vi "Set temperature.vi"(8 "error in (no error)":errorcluster, 9 "Heater":T1, 10 "Temperature":i32, 11 "VISA resource name":refnum<visa-resource-name>) -> (0 "error out":errorcluster, 3 "VISA resource name out":refnum<visa-resource-name>)   [LabVIEW 2020, in "Marlin Instrument Driver.lvlib"]
doc: "Returns the current state of the configured X, Y, Z endstops. Takes into account any 'inverted endstop' settings, so one can confirm that the machine is interpreting the endstops correctly."
uses:
  <instrlib>/Marlin Instrument Driver/Marlin Instrument Driver.lvlib
  <instrlib>/Marlin Instrument Driver/Public/controls/heater.ctl
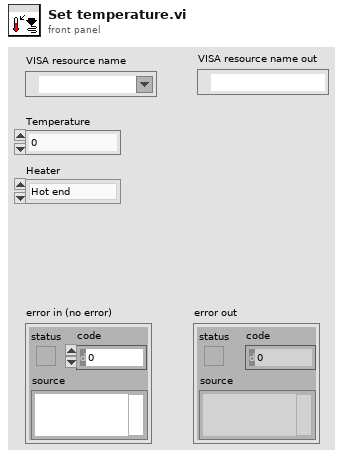
[diagram p1: front panel]
types:
  T1 = typedef "Marlin Instrument Driver.lvlib/heater.ctl" = enum16{"Hot end", "Bed", "Chamber"}
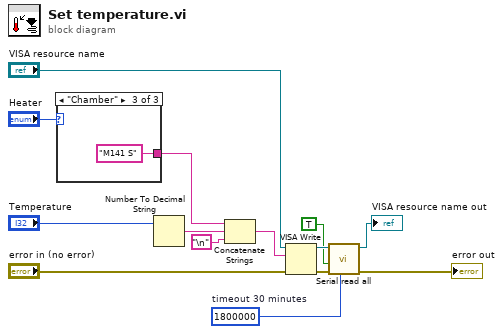
[diagram p0: block diagram]
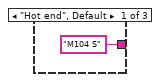
[diagram p2: hidden frame]
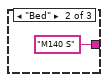
[diagram p3: hidden frame]
diagram:
  w6 = u32 1800000  # timeout 30 minutes
  n1 = case shown="\"Chamber\"" "Heater" {
    tunnel: ["M104 S" "M140 S" "M141 S"] -> w3
    frame "Hot end", Default {
    }
    frame "Bed" {
    }
    frame "Chamber" {
    }
  }
  n2 = Number To Decimal String(number="Temperature") -> (decimal integer string=w1:string)  [unwired: 1 in]
  n3 = Concatenate Strings(w3, w1, "\n") -> (w12:string)
  n4 = VISA Write(VISA resource name="VISA resource name", write buffer=w12, error in (no error)="error in (no error)") -> (VISA resource name out=w10:refnum<visa-resource-name>, error out=w11:errorcluster)  [unwired: 1 out]
  n5 = call <instrlib>:"Serial read all.vi"("timeout (10000ms)"=w6, "error in (no error)"=w11, "Wait for OK"=TRUE, "VISA Refnum in"=w10) -> ("error out"=→"error out":errorcluster, "VISA Refnum out"=→"VISA resource name out":refnum<visa-resource-name>)  [unwired: 4 in, 2 out]
